vi "Prompt for Custom Filter.vi"(6 "Calling VI in":refnum<vi>, 8 "error in (no error)":errorcluster, 11 "Filter Info":T1={"Filter Column"=enum."Description", "Filter Type"=enum."Contains", "Filter Value"="", "New Data?"=FALSE, "Case Sensitive?"=FALSE, "Enabled?"=FALSE}) -> (0 "error out":errorcluster, 2 "OK?":bool, 3 "Filter Info out":T1={"Filter Column"=enum."Description", "Filter Type"=enum."Contains", "Filter Value"="", "New Data?"=FALSE, "Case Sensitive?"=FALSE, "Enabled?"=FALSE})   [LabVIEW 2020, in "VI Properties Editor.lvlib"]
doc: "Displays a window to add a custom filter."
uses:
  VI Properties Editor.lvlib
  CTLs/Filter Column.ctl
  CTLs/Filter Type.ctl
  CTLs/Filter Info.ctl
panel:
  in  "Case Sensitive?":bool caption="Case sensitive"
  in  "Cancel":bool
  in  "OK":bool
  in  "Filter Type Enum":T3
  in  "Filter Type":u16(ring) items=["Contains", "Equals", "Starts with", "Ends with", "Does not contain", "Does not equal", "Is empty", "Is not empty"]
  in  "Filter Column":u16(ring) items=["Name", "Path", "Type", "Window Title", "Description", "Help Path", "Help Tag", "Custom Title?", "Reentrant?", "Inlined?"]
  in  "Filter Value":string
  in  "Filter Column Enum":T2
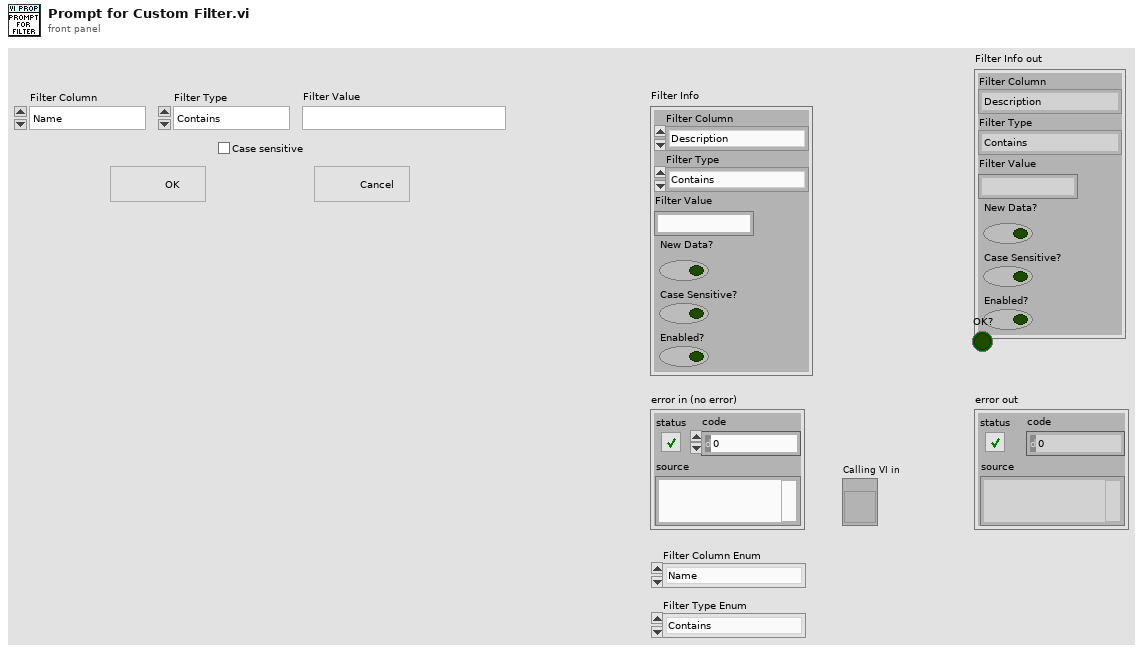
[diagram p1: front panel]
types:
  T1 = typedef "VI Properties Editor.lvlib/Filter Info.ctl" = cluster{"Filter Column":T2, "Filter Type":T3, "Filter Value":string, "New Data?":bool, "Case Sensitive?":bool, "Enabled?":bool}
  T2 = typedef "VI Properties Editor.lvlib/Filter Column.ctl" = enum16{"Name", "Path", "Type", "Window Title", "Description", "Help Path", "Help Tag", "Custom Title?", "Reentrancy", "Inlined?", "Help URL", "Help Type", "Allow Debugging?", "Auto Error Handling?", "Run When Opened?", "Suspend When Called?", "Priority", "Preferred Exec Sytem", "Control Label", "Control Caption", "Control Description", "Control Tip Strip"}
  T3 = typedef "VI Properties Editor.lvlib/Filter Type.ctl" = enum16{"Contains", "Equals", "Starts with", "Ends with", "Is empty", "Does not contain", "Does not equal", "Is not empty"}
  T4 = enum32{"Invalid", "Standard", "Closed", "Hidden", "Minimized", "Maximized"}
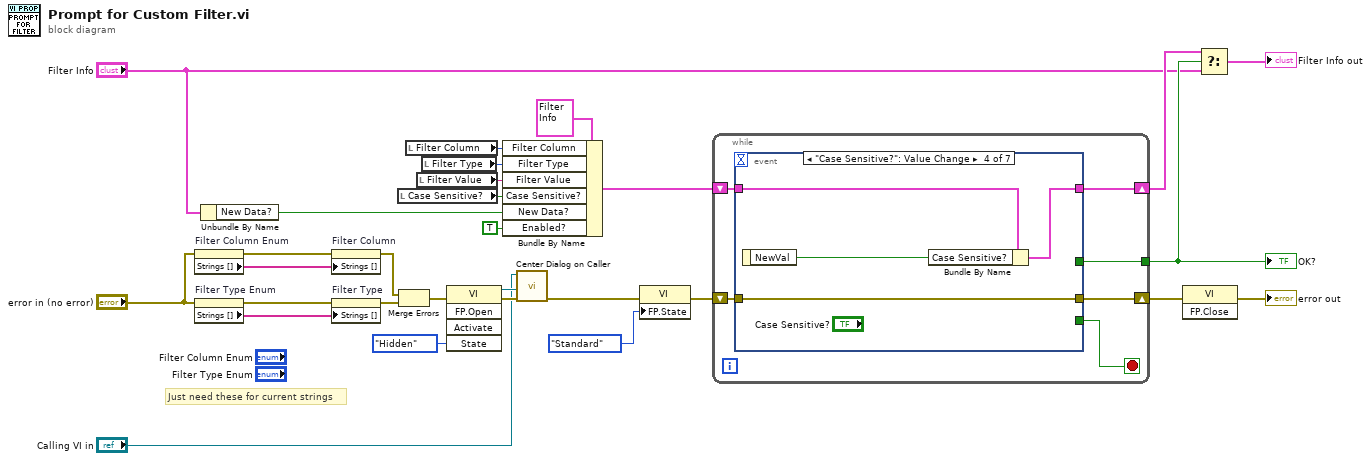
[diagram p0: block diagram]
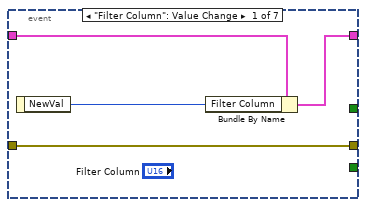
[diagram p2: hidden frame]
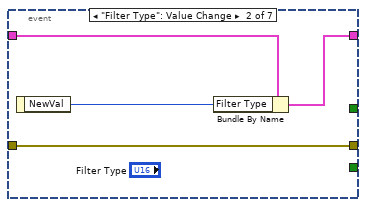
[diagram p3: hidden frame]
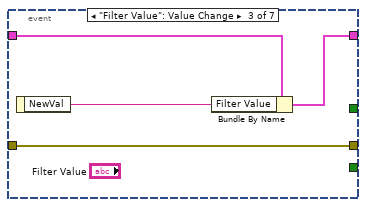
[diagram p4: hidden frame]
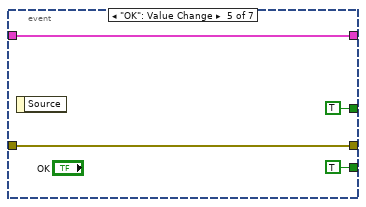
[diagram p5: hidden frame]
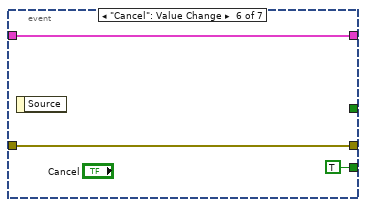
[diagram p6: hidden frame]
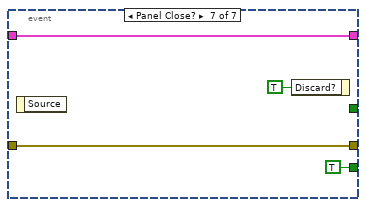
[diagram p7: hidden frame]
diagram:
  # "Just need these for current strings"
  n1 = property on="Filter Column Enum" class="Enum (strict)"(error in="error in (no error)") -> (error out=w27:errorcluster, "Strings []"=w29:string[])  [unwired: 1 in, 1 out]
  n2 = property on="Filter Type Enum" class="Enum (strict)"(error in="error in (no error)") -> (error out=w26:errorcluster, "Strings []"=w28:string[])  [unwired: 1 in, 1 out]
  n3 = Unbundle By Name("Filter Info") -> ("New Data?"=w10:bool)
  n4 = property on="Filter Column" class="Ring (strict)"(error in=w27, "Strings []"=w29) -> (error out=w25:errorcluster)  [unwired: 1 in, 1 out]
  n5 = property on="Filter Type" class="Ring (strict)"(error in=w26, "Strings []"=w28) -> (error out=w24:errorcluster)  [unwired: 1 in, 1 out]
  n6 = local read "Case Sensitive?"() -> (w1:bool)
  n7 = Merge Errors(w25, w24) -> (w3:errorcluster)
  n8 = local read "Filter Column"() -> (w13:u16)
  n9 = local read "Filter Value"() -> (w14:string)
  n10 = local read "Filter Type"() -> (w12:u16)
  n11 = invoke class="VI" method="FP.Open"(error in=w3, "State"=T4."Hidden") -> (reference out=w6:refnum<vi>, error out=w7:errorcluster)  [unwired: 3 in, 3 out]
  n12 = Bundle By Name(cluster=T1 {"Filter Column"=enum."Description", "Filter Type"=enum."Contains", "Filter Value"="", "New Data?"=FALSE, "Case Sensitive?"=FALSE, "Enabled?"=FALSE} ("Filter Info"), "Filter Column"=w13, "Filter Type"=w12, "Filter Value"=w14, "Case Sensitive?"=w1, "New Data?"=w10, "Enabled?"=TRUE) -> (w17:T1)
  n13 = call "Center Dialog on Caller.vi"("error in (no error)"=w7, "Dialog VI"=w6, "Calling VI in"="Calling VI in") -> ("error out"=w9:errorcluster)  [unwired: 7 in, 1 out]
  n14 = property class="VI"(error in=w9, "FP.State"=T4."Standard" ("Front Panel Window:State")) -> (error out=w2:errorcluster)  [unwired: 1 in, 1 out]
  n15 = while {
    tunnel: [w30] -> w20
    shift-right: [w34] -> w19
    shift-left: w17 -> [w35]
    shift-right: [w32] -> w23
    shift-left: w2 -> [w33]
    stop <- w31 stop-if-true
    n16 = event shown="[3] \"Case Sensitive?\": Value Change" {
      selector: _ -> [_ _ _ _ _ _ _]
      dyn-events: _ -> [_ _ _ _ _ _ _]
      timeout: _ -> [_ _ _ _ _ _ _]
      tunnel: w35 -> [w39 w43 w47 w51 w52 w56 w59]
      tunnel: [w37 w41 w45 w49 w52 w56 w59] -> w34
      tunnel: w33 -> [w36 w40 w44 w48 w55 w58 w62]
      tunnel: [w36 w40 w44 w48 w55 w58 w62] -> w32
      tunnel: [_ _ _ _ TRUE TRUE TRUE] -> w31
      tunnel: [_ _ _ _ TRUE _ _] -> w30
      event "Filter Column": Value Change {
        n17 = event-data() -> ("NewVal"=w38:u16)  [unwired: 1 in]
        n18 = Bundle By Name(cluster=w39, "Filter Column"=w38) -> (w37:T1)
      }
      event "Filter Type": Value Change {
        n19 = event-data() -> ("NewVal"=w42:u16)  [unwired: 1 in]
        n20 = Bundle By Name(cluster=w43, "Filter Type"=w42) -> (w41:T1)
      }
      event "Filter Value": Value Change {
        n21 = event-data() -> ("NewVal"=w46:string)  [unwired: 1 in]
        n22 = Bundle By Name(cluster=w47, "Filter Value"=w46) -> (w45:T1)
      }
      event "Case Sensitive?": Value Change {
        n23 = event-data() -> ("NewVal"=w50:bool)  [unwired: 1 in]
        n24 = Bundle By Name(cluster=w51, "Case Sensitive?"=w50) -> (w49:T1)
      }
      event "OK": Value Change {
        n25 = event-data() -> ()  [unwired: 1 in, 1 out]
      }
      event "Cancel": Value Change {
        n26 = event-data() -> ()  [unwired: 1 in, 1 out]
      }
      event Panel Close? {
        n27 = event-data() -> ()  [unwired: 1 in, 1 out]
        n28 = event-data("Discard?"=TRUE) -> ()  [unwired: 1 in, 1 out]
      }
    }
  }
  "OK?" <- w20
  n29 = invoke class="VI" method="FP.Close"(error in=w23) -> (error out=→"error out":errorcluster)  [unwired: 2 in, 2 out]
  n30 = Select(t=w19, s=w20, f="Filter Info") -> (s? t:f=→"Filter Info out":T1)
